vi "niRFUtil WFM Aggregate Waveforms (complex wfm).vi"(2 "Default Value (0)":sgl min=0 max=127 format="%.2f", 3 "WFM replace mode":T1, 4 "Waveforms In":T2[](array[typedef]) {"y" format="%.2f"; "dx" format="%^.2e"; "x0" format="%^.2e"}) -> (1 "Waveform Out":T2 {"y" format="%.2f"; "dx" format="%^.2e"; "x0" format="%^.2e"})   [LabVIEW 2015, in "niRFUtil.lvlib"]
doc: "(c) Copyright 2006, National Instruments, Inc. This VI may not be duplicated, sold, or distributed without written consent from National Instruments."
uses:
  niRFUtil.lvlib
  Includes/niRFUtil INC Complex Waveform.ctl
  Includes/niRFUtil INC Complex Array.ctl
  Includes/niRFUtil INC Waveform Replace Mode.ctl
  niRFUtil WFM Replace Waveform Segment (complex wfm).vi
  Measurements/niRFUtil MEAS Waveform Statistics (complex wfm).vi
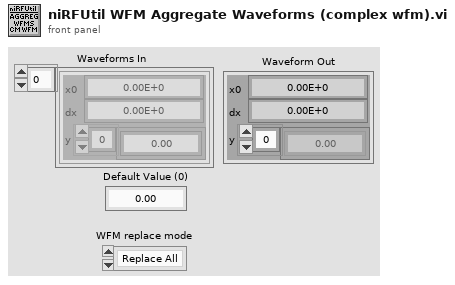
[diagram p1: front panel]
types:
  T1 = typedef "niRFUtil.lvlib/niRFUtil INC Waveform Replace Mode.ctl" = enum16{"Replace All", "Replace Pt By Pt"}
  T2 = typedef "niRFUtil.lvlib/niRFUtil INC Complex Waveform.ctl" = cluster{"x0":dbl, "dx":dbl, "y":T3}
  T3 = typedef "niRFUtil.lvlib/niRFUtil INC Complex Array.ctl" = csg[]
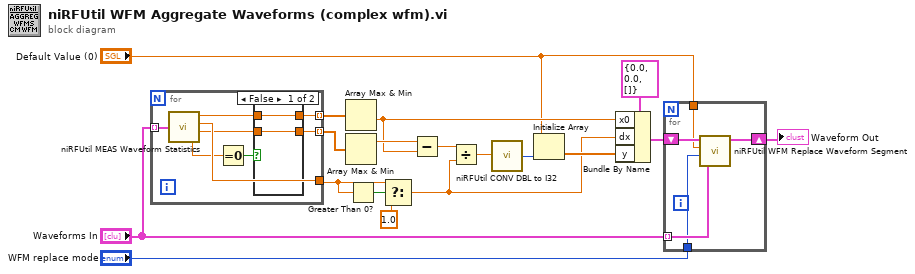
[diagram p0: block diagram]
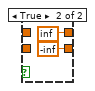
[diagram p2: hidden frame]
diagram:
  n1 = for {
    tunnel: "Waveforms In" -> [w25] mode=indexing
    tunnel: [w22] -> w18 mode=indexing
    tunnel: [w21] -> w17 mode=indexing
    tunnel: [w26] -> w11
    n2 = call-poly "niRFUtil MEAS Waveform Statistics.vi"("Waveform In"=w25) -> ("Start"=w24:dbl, "Interval"=w26:dbl, "End + Interval"=w23:dbl, "Duration"=w20:dbl)  [unwired: 4 in]
    n3 = Equal To 0?(x=w20) -> (x = 0?=w19:bool)
    n4 = case shown="False" w19 {
      tunnel: w24 -> [w28 _]
      tunnel: w23 -> [w27 _]
      tunnel: [w28 inf] -> w22
      tunnel: [w27 -inf] -> w21
      frame False {
      }
      frame True {
      }
    }
  }
  n5 = Array Max & Min(array=w18) -> (min value=w6:dbl)  [unwired: 3 out]
  n6 = Array Max & Min(array=w17) -> (max value=w9:dbl)  [unwired: 3 out]
  n7 = Greater Than 0?(x=w11) -> (x > 0?=w12:bool)
  n8 = Select(t=w11, s=w12, f=1.0) -> (s? t:f=w8:dbl)
  n9 = Subtract(x=w9, y=w6) -> (x-y=w5:dbl)
  n10 = Divide(x=w5, y=w8) -> (x/y=w4:dbl)
  n11 = call "niRFUtil CONV DBL to I32.vi"("Numeric (DBL)"=w4) -> ("Numeric (I32)"=w3:i32)  [unwired: 14 in]
  n12 = Initialize Array("Default Value (0)", w3) -> (w16:sgl[])
  n13 = Bundle By Name(cluster=T2 {"x0"=0.0, "dx"=0.0, "y"=[]} ("Complex Waveform"), "x0"=w6, "dx"=w8, "y"=w16) -> (w14:T2)
  n14 = for {
    shift-right: [w33] -> w7
    shift-left: w14 -> [w35]
    tunnel: "Waveforms In" -> [w34] mode=indexing
    tunnel: "WFM replace mode" -> [w32]
    tunnel: "Default Value (0)" -> [w31]
    n15 = call-poly "niRFUtil WFM Replace Waveform Segment.vi"("Waveform Segment"=w34, "WFM replace mode"=w32, "Default Value (0)"=w31, "Waveform In"=w35) -> ("Waveform Out"=w33:T2)  [unwired: 3 in]
  }
  "Waveform Out" <- w7
